vi "PXI-Default Config.vi"(0 "ExternalTrigger":bool, 4 "MaxPresentations":i32=1000000, 7 "error in (no error)":errorcluster, 8 "Auto Ramping?":bool, 12 "Ramping Parameters":T2={"Ramp up?"=FALSE, "Ramp down?"=FALSE, "Ramp duration (msecs)"=5.0, "Ramp type"=enum."Cos2"}) -> (27 "error out":errorcluster)   [LabVIEW 2020]
uses:
  Type Defs/Ramping Params.ctl
  Type Defs/Channel Struct.ctl
  DAQ Engine VIs/PXI Globals.vi
panel:
  in  "External Start":bool
  in  "DO Config":bool
  in  "DI Config":bool
  in  "AO DoubleBuffering":bool=TRUE
  in  "AO Gain (Property Node)":dbl[](array[slide])=[0.0, 0.0, 0.0, -4.440892098500626e-16, 0.0, 0.0, 0.0, 0.0, 0.0, 0.0] min=-40.0 max=0.0 step=20.0 scale format="%#_2g"
  in  "Bypass NEB":bool
  in  "Stop on MaxPresentations":bool
  in  "Reload Signal Bank":enum32{"OFF", "ENABLED", "FORCED"}(radio)=enum."ENABLED"
  in  "AI BufferSize":i32=10000
  in  "# of extra buffers":i32=2
  in  "TCPData":bool
  in  "Clear Output Channels Cluster":T1={"AO1"=TRUE, "AO2"=FALSE, "AO3"=TRUE, "AO4"=FALSE, "AO5"=FALSE, "AO6"=FALSE, "AO7"=FALSE, "AO8"=FALSE, "AO9"=FALSE, "AO10"=FALSE}
  in  "RouteSyncTaskSampleClk":bool
  in  "BufferSize":i32=10000
  in  "Send Data":bool=TRUE
  in  "AO BufferReWrite":bool=TRUE
  in  "AO ClearTasks":bool=TRUE
  in  "Counter ClearTask":bool=TRUE
  in  "AI ClearTasks":bool=TRUE
  in  "Counter Config":bool
  in  "AO Config":bool
  in  "AI Config":bool
  # "1"
  # "2"
  # "3"
  # "4"
  # "5"
  # "6"
  # "7"
  # "8"
  # "9"
  # "10"
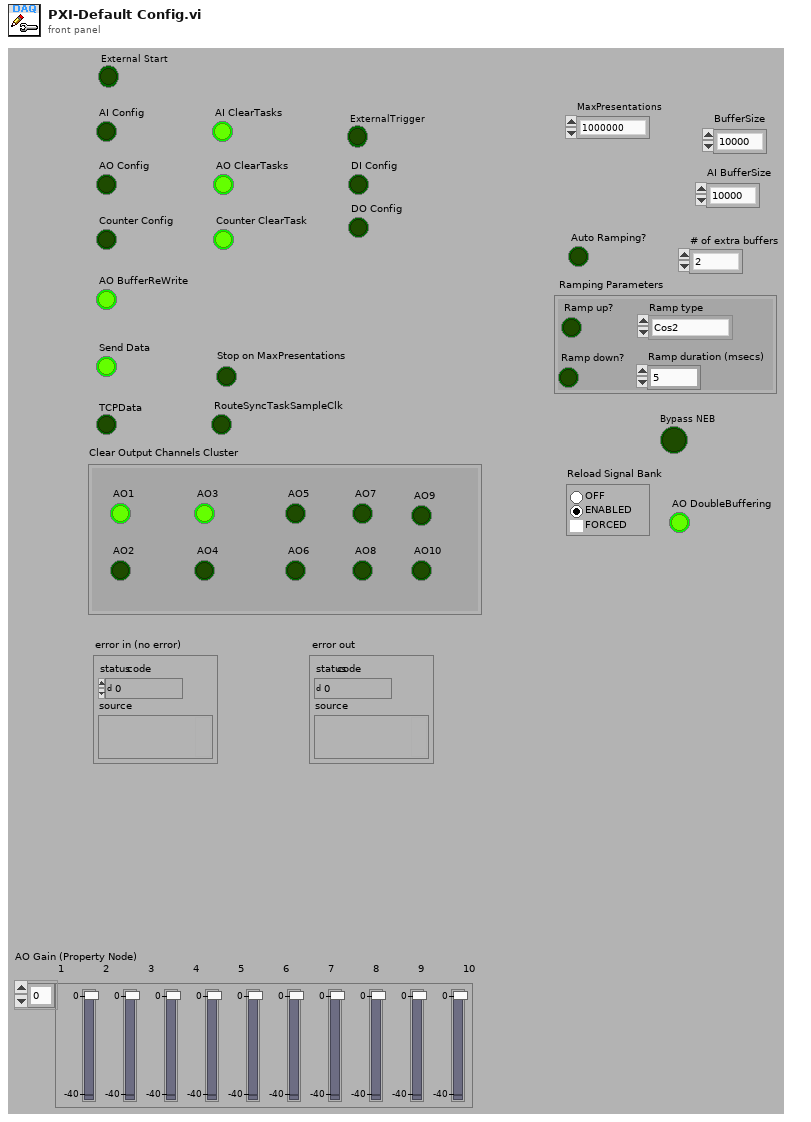
[diagram p1: front panel]
types:
  T1 = cluster{"AO1":bool, "AO2":bool, "AO3":bool, "AO4":bool, "AO5":bool, "AO6":bool, "AO7":bool, "AO8":bool, "AO9":bool, "AO10":bool}
  T2 = typedef "Ramping Params.ctl" = cluster{"Ramp up?":bool, "Ramp down?":bool, "Ramp duration (msecs)":dbl, "Ramp type":enum16{"Linear", "Cos2"}}
  T3 = enum16{"Init", "Write", "Read", "Latch setup", "Compute comp."}
  T4 = typedef "Channel Struct.ctl" = cluster{"Channel name":string, "Vmax":dbl, "Vmin":dbl, "Rate":dbl, "Terminal configuration":i32, "Physical Channel":tag, "Regenerate":bool}
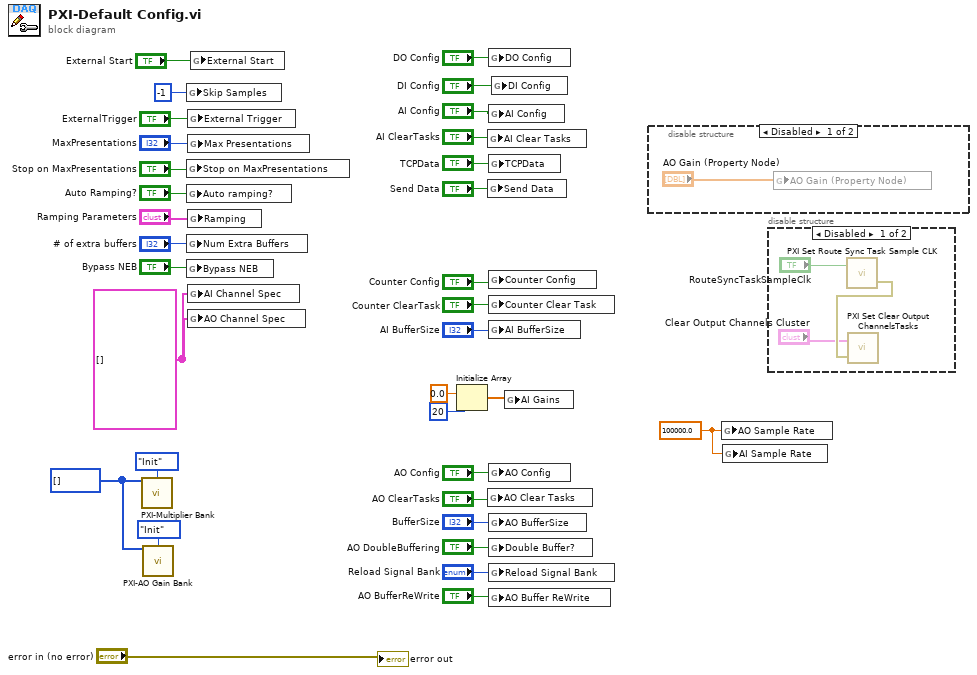
[diagram p0: block diagram]
diagram:
  w3 = 100000.0 ("AO Sample Rate")
  w9 = i32[] [] ("AO Channels")
  w32 = T4[] [] ("AI Channel Spec")
  n1 = call "PXI-Multiplier Bank.vi"("AO Channels"=w9, "Action"=enum16{"Init", "Write", "Read"}."Init") -> ()  [unwired: 11 in, 3 out]
  n2 = call "PXI-AO Gain Bank.vi"("AO Channels"=w9, "Action"=T3."Init") -> ()  [unwired: 8 in, 6 out]
  n3 = global write "PXI Globals.vi" "Skip Samples"(-1 ("Skip Samples")) -> ()
  n4 = global write "PXI Globals.vi" "Stop on MaxPresentations"("Stop on MaxPresentations") -> ()
  n5 = global write "PXI Globals.vi" "Auto ramping?"("Auto Ramping?") -> ()
  n6 = global write "PXI Globals.vi" "Num Extra Buffers"("# of extra buffers") -> ()
  n7 = global write "PXI Globals.vi" "Bypass NEB"("Bypass NEB") -> ()
  n8 = global write "PXI Globals.vi" "External Trigger"("ExternalTrigger") -> ()
  n9 = global write "PXI Globals.vi" "Max Presentations"("MaxPresentations") -> ()
  n10 = global write "PXI Globals.vi" "Ramping"("Ramping Parameters") -> ()
  n11 = global write "PXI Globals.vi" "AI Channel Spec"(w32) -> ()
  n12 = global write "PXI Globals.vi" "AO Channel Spec"(w32) -> ()
  n13 = global write "PXI Globals.vi" "External Start"("External Start") -> ()
  n14 = Initialize Array(0.0 ("element"), 20 ("dimension size")) -> (w7:dbl[])
  n15 = global write "PXI Globals.vi" "AI Clear Tasks"("AI ClearTasks") -> ()
  n16 = global write "PXI Globals.vi" "Send Data"("Send Data") -> ()
  n17 = global write "PXI Globals.vi" "AO Clear Tasks"("AO ClearTasks") -> ()
  n18 = global write "PXI Globals.vi" "DO Config"("DO Config") -> ()
  n19 = global write "PXI Globals.vi" "AI Config"("AI Config") -> ()
  n20 = global write "PXI Globals.vi" "TCPData"("TCPData") -> ()
  n21 = global write "PXI Globals.vi" "Counter Config"("Counter Config") -> ()
  n22 = global write "PXI Globals.vi" "Counter Clear Task"("Counter ClearTask") -> ()
  n23 = global write "PXI Globals.vi" "AI BufferSize"("AI BufferSize") -> ()
  n24 = global write "PXI Globals.vi" "AO Config"("AO Config") -> ()
  n25 = global write "PXI Globals.vi" "AO BufferSize"("BufferSize") -> ()
  n26 = global write "PXI Globals.vi" "Double Buffer?"("AO DoubleBuffering") -> ()
  n27 = global write "PXI Globals.vi" "Reload Signal Bank"("Reload Signal Bank") -> ()
  n28 = global write "PXI Globals.vi" "AO Buffer ReWrite"("AO BufferReWrite") -> ()
  n29 = global write "PXI Globals.vi" "DI Config"("DI Config") -> ()
  n30 = global write "PXI Globals.vi" "AI Gains"(w7) -> ()
  n31 = disable-structure shown="Disabled" {
    frame Disabled {
      n32 = global write "PXI Globals.vi" "AO Gain (Property Node)"("AO Gain (Property Node)") -> ()
    }
    frame Enabled {
    }
  }
  n33 = global write "PXI Globals.vi" "AO Sample Rate"(w3) -> ()
  n34 = global write "PXI Globals.vi" "AI Sample Rate"(w3) -> ()
  n35 = disable-structure shown="Disabled" {
    frame Disabled {
      n36 = call "PXI Set Route Sync Task Sample CLK.vi"("RouteSyncTaskSampleClk"="RouteSyncTaskSampleClk") -> ("error out"=w36:errorcluster)  [unwired: 2 in]
      n37 = call "PXI Set Clear Output ChannelsTasks.vi"("error in (no error)"=w36, "Clear Output Channels Cluster"="Clear Output Channels Cluster") -> ()  [unwired: 1 in, 1 out]
    }
    frame Enabled {
    }
  }
  "error out" <- "error in (no error)"
